vi "SubVI_Filter_EEG.vi"(6 "high cutoff freq":dbl=1.0, 8 "error in (no error)":errorcluster, 9 "Interpolant Size":dbl, 10 "Resampling rate":dbl, 11 "Clean EEG In":T1) -> (0 "error out":errorcluster, 3 "Filtered EEG Out":T1)   [LabVIEW 2020]
uses:
  <extravilib>/ChannelInstances/Stream-a[.,.](dbl)/)Channel.ctl
  <vilib>/Analysis/3filter.llb/Filter Passband Type.ctl
  <extravilib>/ChannelInstances/Stream-a[.,.](dbl)/EndpointRead.vi
  <extravilib>/ChannelInstances/Stream-a[.,.](dbl)/Endpoint.vi
  Global 1.vi
  <extravilib>/ChannelInstances/Stream-a[.,.](dbl)/)Channel.vi
  <resource>/ChannelSupport/_ChannelSupport/WaitIfNeeded.vi
  <vilib>/Analysis/NI_AALBase.lvlib
  <vilib>/ptbypt/NI_PtbyPt.lvlib
  <extravilib>/ChannelInstances/Stream-a[.,.](dbl).lvlib
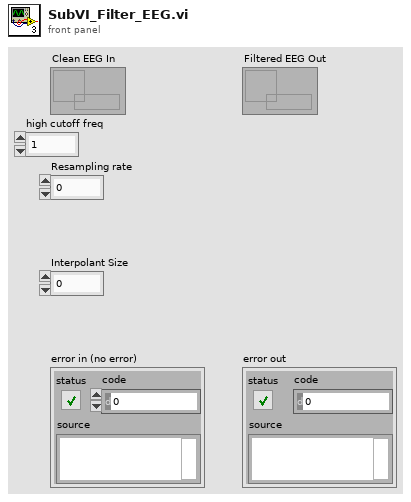
[diagram p1: front panel]
types:
  T1 = typedef "Stream-a[.,.](dbl).lvlib/)Channel.ctl" = refnum<queue>
  T2 = typedef "NI_AALBase.lvlib/Filter Passband Type.ctl" = enum32{"Lowpass", "Highpass", "Bandpass", "Bandstop"}
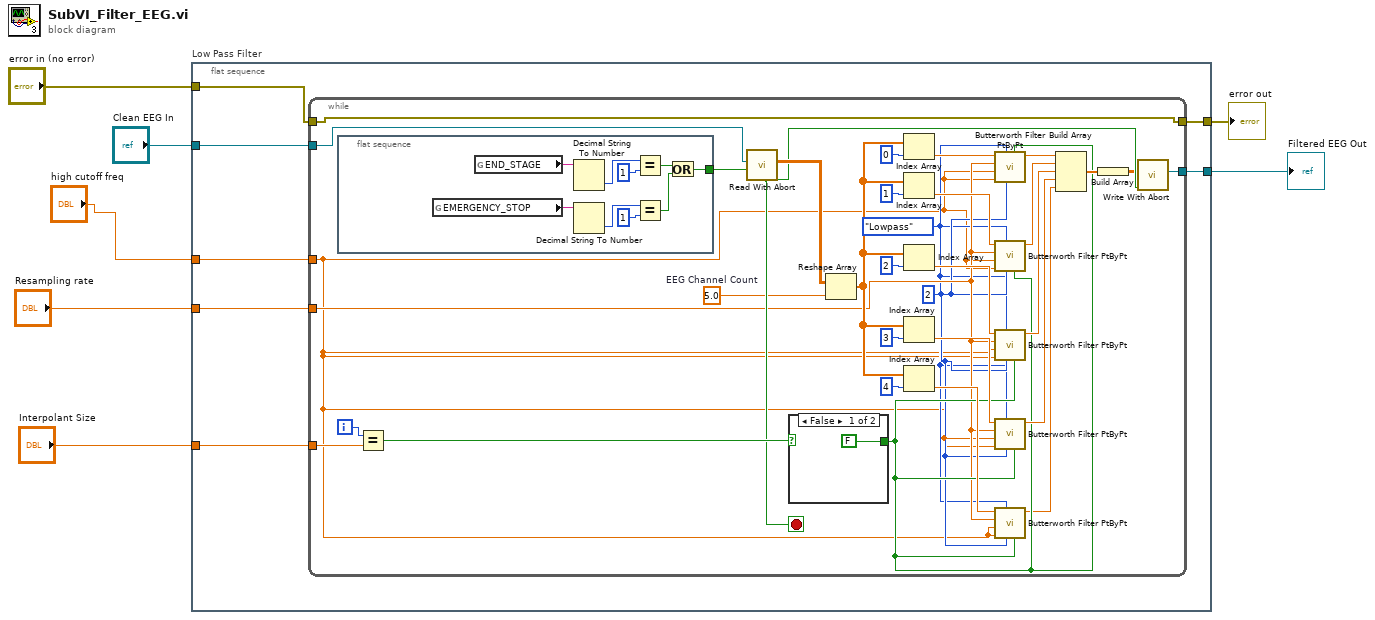
[diagram p0: block diagram]
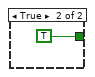
[diagram p2: hidden frame]
diagram:
  n1 = flat-sequence "Low Pass Filter" {
    tunnel: "Clean EEG In" -> [w14]
    tunnel: [w13] -> w3
    tunnel: "Interpolant Size" -> [w12]
    tunnel: "Resampling rate" -> [w11]
    tunnel: "error in (no error)" -> [w10]
    tunnel: [w9] -> w4
    tunnel: "high cutoff freq" -> [w8]
    frame #0 {
      n2 = while {
        tunnel: w14 -> [w34]
        tunnel: [w32] -> w13
        tunnel: w12 -> [w30]
        tunnel: w11 -> [w23]
        tunnel: w10 -> [w16]
        tunnel: [w16] -> w9
        tunnel: w8 -> [w15]
        i -> [w31]
        stop <- w28 stop-if-true
        w19 = 5.0  # EEG Channel Count
        w22 = 2 ("order")
        w21 = Filter_Passband_Type."Lowpass" ("filter type")
        n3 = flat-sequence {
          tunnel: [w48] -> w17
          frame #0 {
            n4 = global read "Global 1.vi" "EMERGENCY_STOP"() -> (w51:string)
            n5 = global read "Global 1.vi" "END_STAGE"() -> (w56:string)
            n6 = Decimal String To Number(string=w56) -> (number=w55:i32)  [unwired: 2 in, 1 out]
            n7 = Decimal String To Number(string=w51) -> (number=w53:i32)  [unwired: 2 in, 1 out]
            n8 = Equal?(x=w55, y=1) -> (x = y?=w49:bool)
            n9 = Equal?(x=w53, y=1) -> (x = y?=w50:bool)
            n10 = Or(x=w49, y=w50) -> (x .or. y?=w48:bool)
          }
        }
        n11 = Equal?(x=w31, y=w30) -> (x = y?=w29:bool)
        n12 = call <extravilib>:"Read With Abort.vi"("abort"=w17, "channel"=w34) -> ("element"=w33:dbl[][], "aborted?"=w28:bool)  [unwired: 4 in, 4 out]
        n13 = case shown="False" w29 {
          tunnel: [FALSE ("init/cont (init:F)") TRUE ("init/cont (init:F)")] -> w24
          frame False {
          }
          frame True {
          }
        }
        n14 = Reshape Array(w33, w19) -> (w25:dbl[])
        n15 = Index Array(array=w25, index=0 ("disabled index (col)")) -> (element=w43:dbl)
        n16 = Index Array(array=w25, index=1 ("disabled index (col)")) -> (element=w44:dbl)
        n17 = Index Array(array=w25, index=2 ("disabled index (col)")) -> (element=w45:dbl)
        n18 = Index Array(array=w25, index=3 ("disabled index (col)")) -> (element=w46:dbl)
        n19 = Index Array(array=w25, index=4 ("disabled index (col)")) -> (element=w27:dbl)
        n20 = call <vilib>:"Butterworth Filter PtByPt.vi"("initialize"=w24, "order"=w22, "filter type"=w21, "low cutoff freq: fl"=w15, "high cutoff freq: fh"=w15, "sampling freq: fs"=w23, "x"=w43) -> ("Filtered x"=w39:dbl)  [unwired: 2 in, 1 out]
        n21 = call <vilib>:"Butterworth Filter PtByPt.vi"("initialize"=w24, "order"=w22, "filter type"=w21, "low cutoff freq: fl"=w15, "high cutoff freq: fh"=w15, "sampling freq: fs"=w23, "x"=w44) -> ("Filtered x"=w40:dbl)  [unwired: 2 in, 1 out]
        n22 = call <vilib>:"Butterworth Filter PtByPt.vi"("initialize"=w24, "order"=w22, "filter type"=w21, "low cutoff freq: fl"=w15, "high cutoff freq: fh"=w15, "sampling freq: fs"=w23, "x"=w45) -> ("Filtered x"=w41:dbl)  [unwired: 2 in, 1 out]
        n23 = call <vilib>:"Butterworth Filter PtByPt.vi"("initialize"=w24, "order"=w22, "filter type"=w21, "low cutoff freq: fl"=w15, "high cutoff freq: fh"=w15, "sampling freq: fs"=w23, "x"=w46) -> ("Filtered x"=w42:dbl)  [unwired: 2 in, 1 out]
        n24 = call <vilib>:"Butterworth Filter PtByPt.vi"("initialize"=w24, "order"=w22, "filter type"=w21, "low cutoff freq: fl"=w15, "high cutoff freq: fh"=w15, "sampling freq: fs"=w23, "x"=w27) -> ("Filtered x"=w20:dbl)  [unwired: 2 in, 1 out]
        n25 = Build Array(w39, w40, w41, w42, w20) -> (w47:dbl[])
        n26 = Build Array(w47) -> (w18:dbl[][])
        n27 = call <extravilib>:"Write With Abort.vi"("abort"=w28, "element"=w18) -> ("channel"=w32:T1)  [unwired: 6 in, 3 out]
      }
    }
  }
  "error out" <- w4
  "Filtered EEG Out" <- w3
